vi "N5700 Config Output On-Off.vi"(4 "Settle (0 mS)":u32, 5 "error":errorcluster, 7 "Output ON":bool, 8 "VISA":refnum<visa-resource-name>) -> (0 "error out":errorcluster, 3 "VISA out":refnum<visa-resource-name>)   [LabVIEW 2020]
doc: "This VI sets the power supply output ON or OFF. \nIf \"Output ON\" is set FALSE, the output will be turned OFF.\n\nThis VI will wait for \"Settle\" milliseconds after setting the output. If unwired, there will be no delay\n\nNote: After a fault shutdown, the output cannot be turned ON until a 'clear fault' is sent"
panel:
  # "Agilent Technologies  \nSeries N5700A\n  DC Power Supplies"
  # "Set Output ON or OFF"
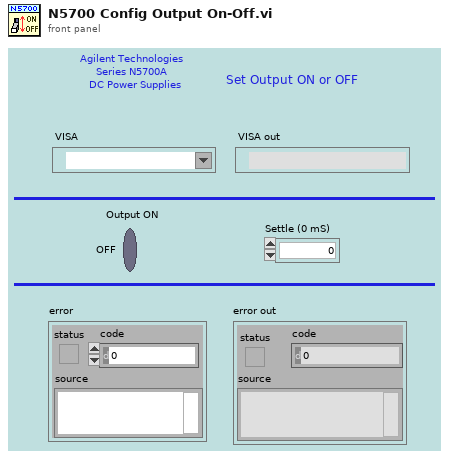
[diagram p1: front panel]
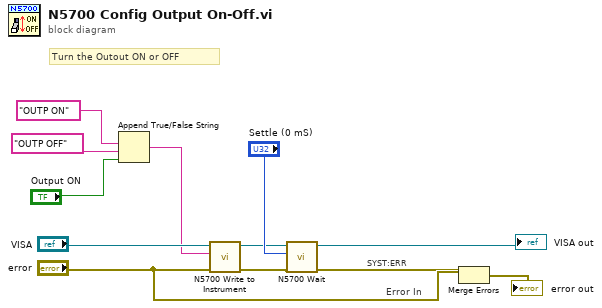
[diagram p0: block diagram]
diagram:
  # "SYST:ERR"
  # "Error In"
  # "Turn the Outout ON or OFF"
  n1 = Append True/False String(1:"Output ON", 2:"OUTP OFF" ("format string"), 3:"OUTP ON" ("format string")) -> (0:w7:string)  [unwired: 1 in]
  n2 = call "N5700 Write to Instrument.vi"("error"="error", "Command"=w7, "VISA"="VISA") -> ("error out"=w5:errorcluster, "VISA out"=w4:refnum<visa-resource-name>)  [unwired: 4 in]
  n3 = call "N5700 Wait.vi"("error"=w5, "Delay (5 mS)"="Settle (0 mS)", "VISA"=w4) -> ("error out"=w2:errorcluster, "VISA out"=→"VISA out":refnum<visa-resource-name>)  [unwired: 4 in]
  n4 = Merge Errors("error", w2) -> (→"error out":errorcluster)
